vi "Save Image.vi"(8 "error in (no error)":errorcluster, 11 "IMAQ Display in":refnum<class "HIJ IMAQdx Display.lvclass">) -> (0 "error out":errorcluster, 2 "Filename":string, 3 "IMAQ Display out":refnum<class "HIJ IMAQdx Display.lvclass">)   [LabVIEW 2020, in "HIJ IMAQdx Display.lvlib" / "HIJ IMAQdx Display.lvclass"]
doc: "Speichert das Kamerabild in PNG Format und ruft Generate Report auf. Wenn Flag \"Time in Filename\" gesetzt ist, wird ein Zeitstempel dem Dateinamen angehängt."
uses:
  HIJ IMAQdx Display.lvclass
  C:/Users/AlexK/work/LabVIEW Programme/POLARIS CAM Log Abw und E/Submodules/HIJ Vision/Display Actors/HIJ Vision Display/HIJ Vision Display/HIJ Vision Display.lvclass
  HIJ Vision Display/HIJ Vision Display/HIJ Vision Display.lvclass/HIJ Vision Display.ctl
  HIJ Vision Display/HIJ Vision Display/Read Image In.vi
  HIJ Vision Display/HIJ Vision Display/Read WorkDir.vi
  HIJ Vision Display/HIJ Vision Display/Read Image Source Name.vi
  HIJ Vision Display/HIJ Vision Display/Read Source in Filename.vi
  HIJ Vision Display/HIJ Vision Display/Read ShotId in Filename.vi
  HIJ Vision Display/HIJ Vision Display/Read ShotID.vi
  HIJ Vision Display/HIJ Vision Display/Read FrameID in Filename.vi
  HIJ Vision Display/HIJ Vision Display/Read TimestampFormat.vi
  HIJ Vision Display/HIJ Vision Display/Read ImageTimeStamp.vi
  HIJ Vision Display/HIJ Vision Display/Read Time in Filename_.vi
  HIJ IMAQdx Display.lvclass/HIJ IMAQdx Display.ctl
  <vilib>/Utility/config.llb/NI_LVConfig.lvlib
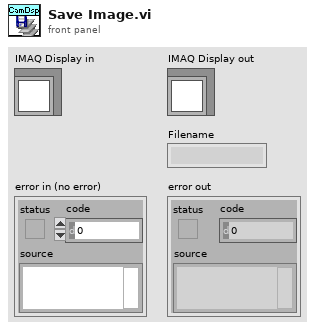
[diagram p1: front panel]
types:
  T1 = typedef "NI_LVConfig.lvlib/Config Data RefNum.ctl" = refnum<k1>
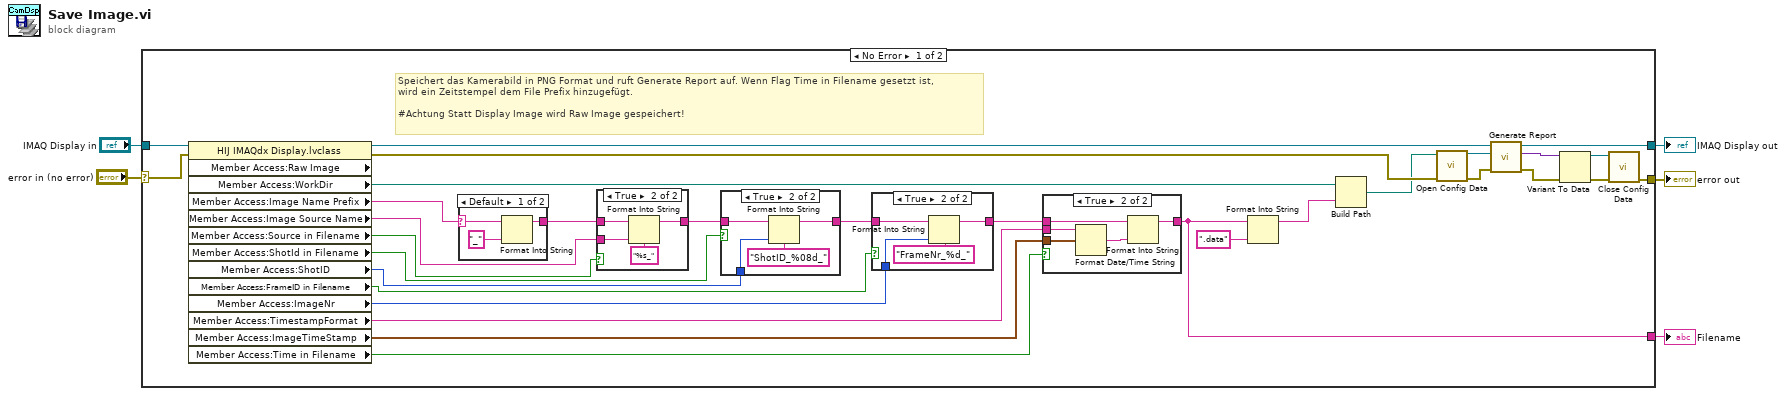
[diagram p0: block diagram]
diagram:
  n1 = case shown="No Error" "error in (no error)" {
    selector: "error in (no error)" -> [w33 w63]
    tunnel: [w22 w63] -> w4
    tunnel: [w27 w62] -> w2
    tunnel: "IMAQ Display in" -> [w35 w62]
    tunnel: [w7 _] -> w1
    frame No Error {
      # "Speichert das Kamerabild in PNG Format und ruft Generate Report auf. Wenn Flag Time in Filename gesetzt ist, \nwird ein Zeitstempel dem File Prefix hinzugefügt.\n\n#Achtung Statt Display Image wird Raw Image gespeichert!"
      n2 = property class="HIJ IMAQdx Display.lvclass" props=["Member Access:Raw Image", "Member Access:WorkDir", "Member Access:Image Name Prefix", "Member Access:Image Source Name", "Member Access:Source in Filename", "Member Access:ShotId in Filename", "Member Access:ShotID", "Member Access:FrameID in Filename", "Member Access:ImageNr", "Member Access:TimestampFormat", "Member Access:ImageTimeStamp", "Member Access:Time in Filename"](reference=w35, error in=w33) -> (reference out=w34:refnum<class "HIJ IMAQdx Display.lvclass">, error out=w36:errorcluster, "Member Access:WorkDir"=w31:path, "Member Access:Image Name Prefix"=w11:string, "Member Access:Image Source Name"=w10:string, "Member Access:Source in Filename"=w9:bool, "Member Access:ShotId in Filename"=w17:bool, "Member Access:ShotID"=w16:i32, "Member Access:FrameID in Filename"=w13:bool, "Member Access:ImageNr"=w14:i32, "Member Access:TimestampFormat"=w21:string, "Member Access:ImageTimeStamp"=w19:timestamp, "Member Access:Time in Filename"=w20:bool)  [unwired: 1 out]
      n3 = case shown="Default" w11 {
        selector: w11 -> [w39 w40]
        tunnel: [w38 w40] -> w8
        frame Default {
          n4 = Format Into String(initial string=w39, "_") -> (resulting string=w38:string)  [unwired: 2 in, 1 out]
        }
        frame "" {
        }
      }
      n5 = case shown="True" w9 {
        tunnel: [w41 w45] -> w12
        tunnel: w8 -> [w41 w44]
        tunnel: w10 -> [_ w43]
        frame False {
        }
        frame True {
          n6 = Format Into String(format string="%s_", initial string=w44, w43) -> (resulting string=w45:string)  [unwired: 1 in, 1 out]
        }
      }
      n7 = case shown="True" w17 {
        tunnel: w12 -> [w46 w50]
        tunnel: [w46 w49] -> w18
        tunnel: w16 -> [_ w48]
        frame False {
        }
        frame True {
          n8 = Format Into String(format string="ShotID_%08d_", initial string=w50, w48) -> (resulting string=w49:string)  [unwired: 1 in, 1 out]
        }
      }
      n9 = case shown="True" w13 {
        tunnel: w18 -> [w51 w55]
        tunnel: [w51 w54] -> w15
        tunnel: w14 -> [_ w52]
        frame False {
        }
        frame True {
          n10 = Format Into String(format string="FrameNr_%d_", initial string=w55, w52) -> (resulting string=w54:string)  [unwired: 1 in, 1 out]
        }
      }
      n11 = case shown="True" w20 {
        tunnel: [w56 w57] -> w7
        tunnel: w15 -> [w56 w59]
        tunnel: w21 -> [_ w61]
        tunnel: w19 -> [_ w58]
        frame False {
        }
        frame True {
          n12 = Format Date/Time String(time format string (%c)=w61, seconds (now)=w58) -> (date/time string=w60:string)  [unwired: 1 in]
          n13 = Format Into String(initial string=w59, w60) -> (resulting string=w57:string)  [unwired: 2 in, 1 out]
        }
      }
      n14 = Format Into String(initial string=w7, ".data" ("format string")) -> (resulting string=w30:string)  [unwired: 2 in, 1 out]
      n15 = Build Path(base path=w31, name or relative path=w30) -> (appended path=w32:path)
      n16 = call <vilib>:"Open Config Data.vi"("error in (no error)"=w36, "configuration file path"=w32) -> ("error out"=w29:errorcluster, "refnum"=w28:T1)  [unwired: 7 in, 1 out]
      n17 = call-dynamic "Generate Report.vi"("error in (no error)"=w29, "Resource In"=w28, "HIJ IMAQdx Display in"=w34) -> ("error out"=w26:errorcluster, "Resource Out"=w24:variant, "HIJ IMAQdx Display out"=w27:refnum<class "HIJ IMAQdx Display.lvclass">)  [unwired: 6 in]
      n18 = Variant To Data(error in=w26, Variant=w24) -> (data=w23:T1, error out=w25:errorcluster)  [unwired: 1 in]
      n19 = call <vilib>:"Close Config Data.vi"("error in (no error)"=w25, "refnum"=w23) -> ("error out"=w22:errorcluster)  [unwired: 8 in, 1 out]
    }
    frame Error {
    }
  }
  "error out" <- w4
  "IMAQ Display out" <- w2
  "Filename" <- w1
